vi "calculate_mag_phase.vi"(3 "periods":u8, 4 "OUT samples":dbl[](array[numeric]), 5 "dt":dbl, 6 "IN samples":dbl[](array[numeric])) -> (0 "Measured Signals":waveform(dbl)[](graph), 1 "Phase":dbl, 2 "Magnitude":dbl)   [LabVIEW 2014]
uses:
  <vilib>/Analysis/4window.llb/windowTd.ctl
  <vilib>/measure/maspectr.llb/FFT Power Spectrum and PSD for 1 Chan.vi
  <vilib>/measure/maspectr.llb/Frequency Response Function (Mag-Phase) 1-1.vi
  <vilib>/measure/NI_MAPro.lvlib
  <vilib>/Analysis/NI_AALPro.lvlib
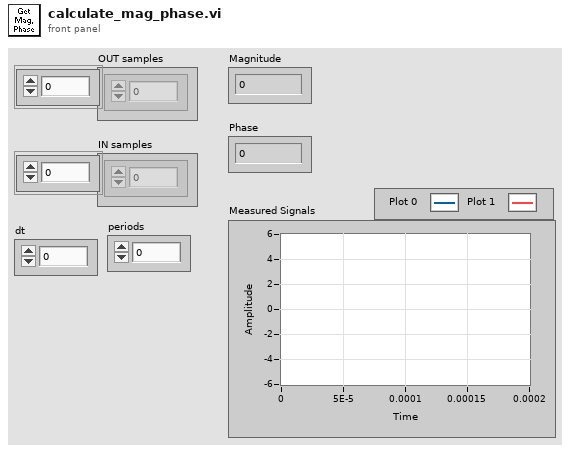
[diagram p1: front panel]
types:
  T1 = typedef "NI_AALPro.lvlib/windowTd.ctl" = u32
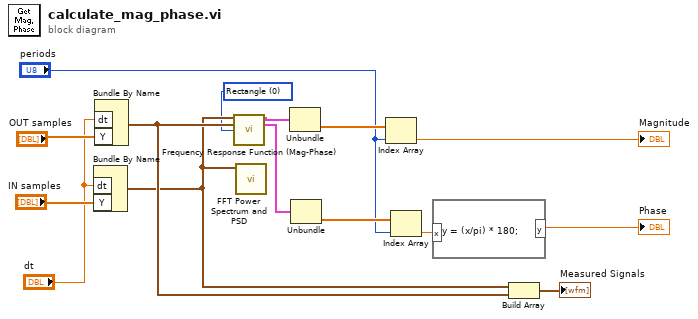
[diagram p0: block diagram]
diagram:
  w5 = T1 0 items=["Rectangle"=0, "Hanning"=1, "Hamming"=2, "Blackman-Harris"=3, "Exact Blackman"=4, "Blackman"=5, "Flat Top"=6, "4 Term B-Harris "=7, "7 Term B-Harris"=8, "Low Sidelobe"=9, "Blackman Nuttall"=11, "Triangle"=30, "Bartlett-Hanning"=31, "Bohman"=32, "Parzen"=33, "Welch"=34, "Kaiser"=60, "Dolph-Chebyshev"=61, "Gaussian"=62] ("window")
  n1 = Bundle By Name("dt"="dt", "Y"="IN samples") -> (w8:waveform(dbl))  [unwired: 1 in]
  n2 = Bundle By Name("dt"="dt", "Y"="OUT samples") -> (w9:waveform(dbl))  [unwired: 1 in]
  n3 = call-poly <vilib>:"Frequency Response Function (Mag-Phase).vi"("time signal X"=w8, "time signal Y"=w9, "window"=w5) -> ("magnitude"=w4:cluster{"f0":dbl, "df":dbl, "magnitude":dbl[]}, "phase"=w6:cluster{"f0":dbl, "df":dbl, "phase":dbl[]})  [unwired: 7 in, 4 out]
  n4 = call-poly <vilib>:"FFT Power Spectrum and PSD.vi"("time signal"=w8) -> ()  [unwired: 7 in, 4 out]
  n5 = Unbundle(w4) -> ("magnitude"=w3:dbl[])  [unwired: 2 out]
  n6 = Unbundle(w6) -> ("phase"=w7:dbl[])  [unwired: 2 out]
  n7 = Index Array(array=w3, index="periods") -> (element=→"Magnitude":dbl)
  n8 = Index Array(array=w7, index="periods") -> (element=w2:dbl)
  n9 = formula code="y = (x/pi) * 180;"("x"=w2) -> ("y"=→"Phase":dbl)
  n10 = Build Array(w8, w9) -> (→"Measured Signals":waveform(dbl)[])
